vi "Cal Aux Corrections.vi"(8 "error in (no error)":errorcluster, 10 "Spectral distribution In":cluster{dbl, dbl}[](graph), 11 "Hardware Resources in":T1) -> (0 "error out":errorcluster, 2 "Spectral distribution Out":cluster{dbl, dbl}[](graph), 3 "Hardware Resources out":T1)   [LabVIEW 2013, in "AvaSpec.lvlib" / "AvaSpec Acquisition.lvlib"]
uses:
  AvaSpec Acquisition.lvlib
  Hardware Configuration.ctl
  Libraries/AS-5216-DLL/AVS settings.ctl
  Sphere Indicator.ctl
  Settings/Measurement Type.ctl
  AvaSpec.lvlib
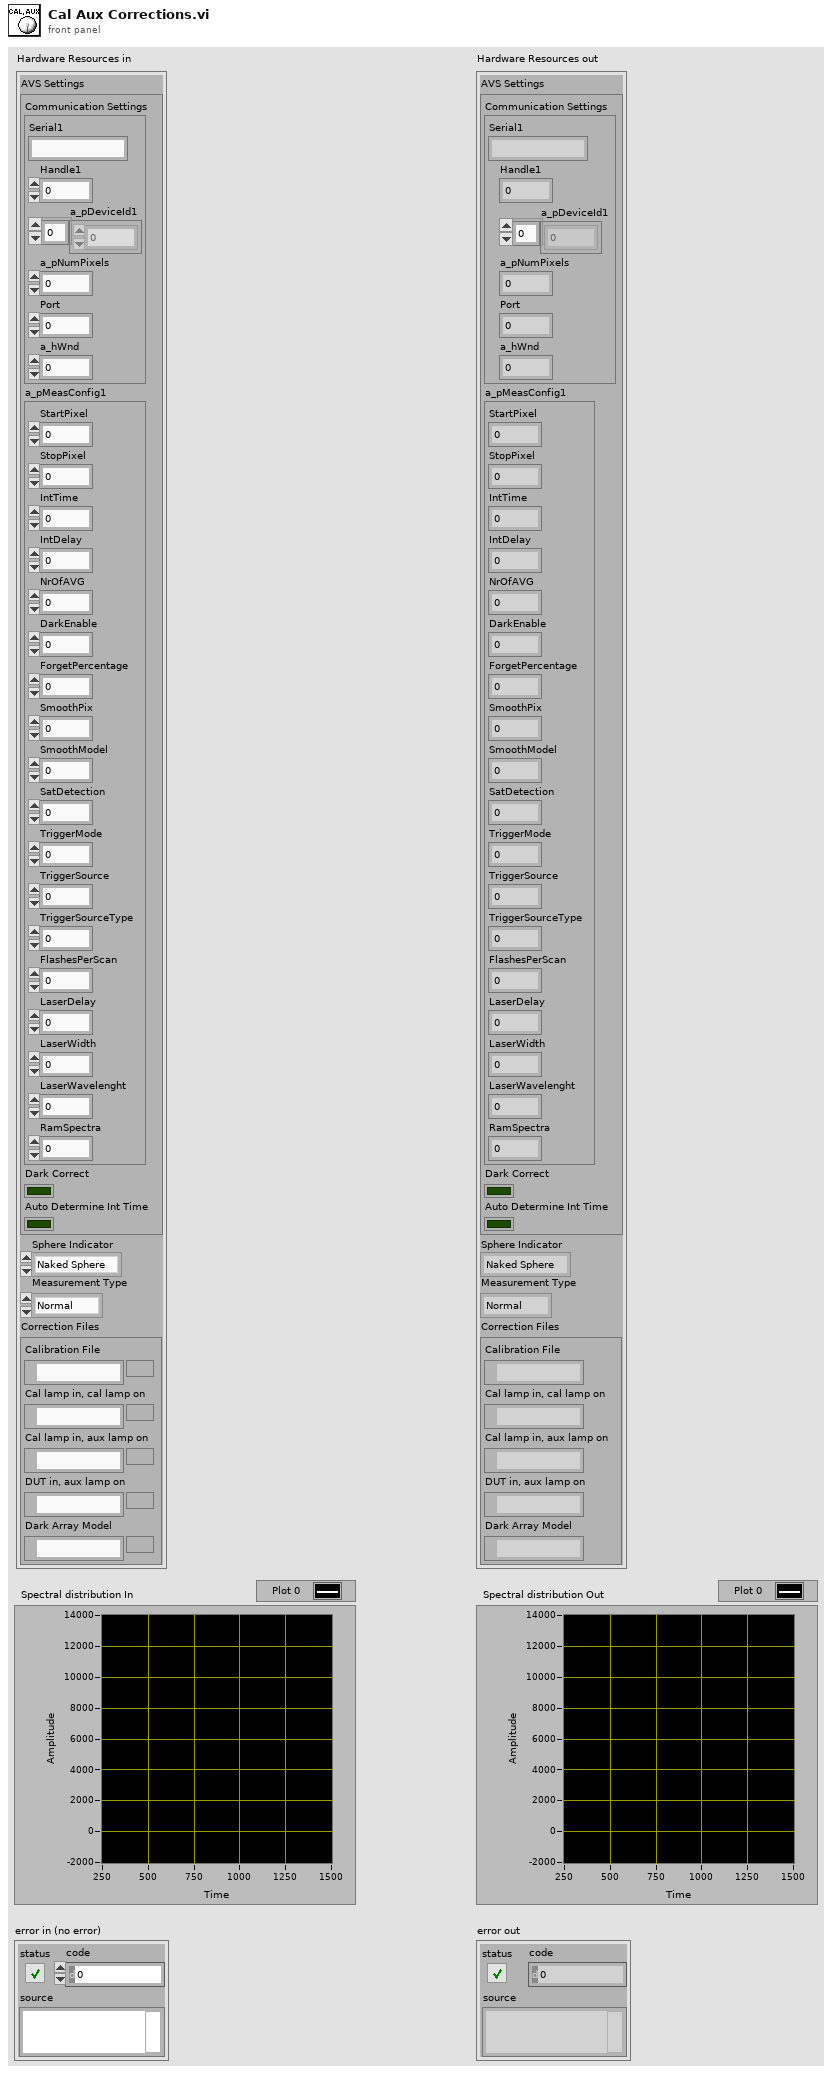
[diagram p1: front panel]
types:
  T1 = typedef "AvaSpec.lvlib/AvaSpec Acquisition.lvlib/Hardware Configuration.ctl" = cluster{"AVS Settings":T2, "Sphere Indicator":T3, "Measurement Type":T4, "Correction Files":cluster{"Calibration File":path, "Cal lamp in, cal lamp on":path, "Cal lamp in, aux lamp on":path, "DUT in, aux lamp on":path, "Dark Array Model":path}}
  T2 = typedef "AvaSpec.lvlib/AVS settings.ctl" = cluster{"Communication Settings":cluster{"Serial1":string, "Handle1":i32, "a_pDeviceId1":u8[], "a_pNumPixels":u16, "Port":i32, "a_hWnd":i32}, "a_pMeasConfig1":cluster{"StartPixel":u16, "StopPixel":u16, "IntTime":sgl, "IntDelay":u32, "NrOfAVG":u32, "DarkEnable":u8, "ForgetPercentage":u8, "SmoothPix":u16, "SmoothModel":u8, "SatDetection":u8, "TriggerMode":u8, "TriggerSource":u8, "TriggerSourceType":u8, "FlashesPerScan":u16, "LaserDelay":u32, "LaserWidth":u32, "LaserWavelenght":sgl, "RamSpectra":u16}, "Dark Correct":bool, "Auto Determine Int Time":bool}
  T3 = typedef "AvaSpec.lvlib/Sphere Indicator.ctl" = enum16{"Naked Sphere", "Insulated Sphere"}
  T4 = typedef "AvaSpec.lvlib/AvaSpec Acquisition.lvlib/Measurement Type.ctl" = enum16{"Normal", "Calibration", "Dark"}
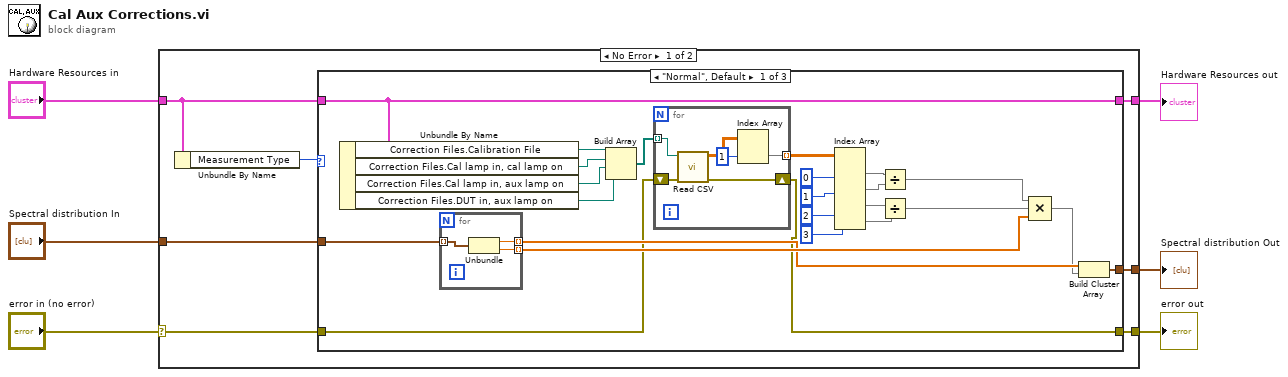
[diagram p0: block diagram]
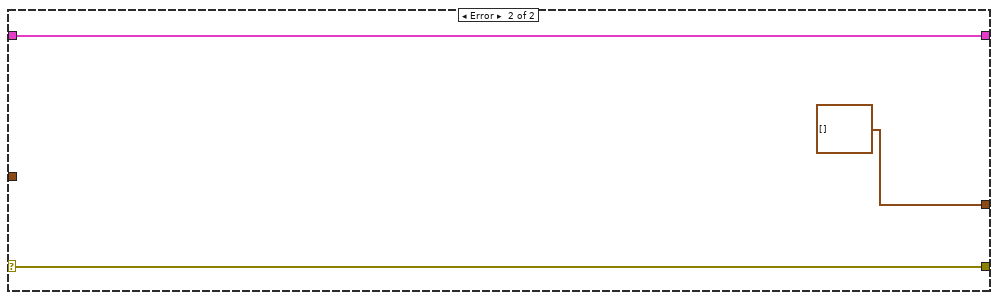
[diagram p4: hidden frame]
diagram:
  n1 = case shown="No Error" "error in (no error)" {
    selector: "error in (no error)" -> [w8 w55]
    tunnel: [w7 w55] -> w5
    tunnel: "Spectral distribution In" -> [w13 _]
    tunnel: "Hardware Resources in" -> [w11 w54]
    tunnel: [w9 w54] -> w2
    tunnel: [w12 cluster{dbl, dbl}[] [] ("Spectral distribution 3")] -> w1
    frame No Error {
      n2 = Unbundle By Name(w11) -> ("Measurement Type"=w10:T4)
      n3 = case shown="\"Normal\", Default" w10 {
        tunnel: w13 -> [w32 w48 w51]
        tunnel: [w23 w48 w51] -> w12
        tunnel: w11 -> [w22 w49 w52]
        tunnel: [w22 w49 w52] -> w9
        tunnel: w8 -> [w15 w47 w50]
        tunnel: [w14 w47 w50] -> w7
        frame "Normal", Default {
          n4 = Unbundle By Name(w22) -> ("Correction Files.Calibration File"=w37:path, "Correction Files.Cal lamp in, cal lamp on"=w36:path, "Correction Files.Cal lamp in, aux lamp on"=w35:path, "Correction Files.DUT in, aux lamp on"=w34:path)
          n5 = for {
            tunnel: w32 -> [w40] mode=indexing
            tunnel: [w39] -> w26 mode=indexing
            tunnel: [w38] -> w25 mode=indexing
            n6 = Unbundle(w40) -> (w38:dbl, w39:dbl)
          }
          n7 = Build Array(w37, w36, w35, w34) -> (w33:path[])
          n8 = for {
            tunnel: w33 -> [w44] mode=indexing
            tunnel: [w45] -> w31 mode=indexing
            shift-right: [w42] -> w14
            shift-left: w15 -> [w41]
            n9 = call "Read CSV.vi"("error in (no error)"=w41, "Path"=w44) -> ("error out"=w42:errorcluster, "all rows"=w43:dbl[][])  [unwired: 7 in, 1 out]
            n10 = Index Array(array=w43, index (col)=1 ("disabled index (col)")) -> (element=w45:dbl[])  [unwired: 1 in]
          }
          n11 = Index Array(array=w31, index (col) #1=0 ("disabled index (col)"), index (col) #2=1 ("index (col)"), index (col) #3=2 ("index (col)"), index (col) #4=3 ("index (col)")) -> (element #1=w21:dbl[], element #2=w20:dbl[], element #3=w19:dbl[], element #4=w18:dbl[])  [unwired: 4 in]
          n12 = Divide(x=w21, y=w20) -> (x/y=w17:dbl[])
          n13 = Divide(x=w19, y=w18) -> (x/y=w16:dbl[])
          n14 = Compound Arithmetic op=MULTIPLY(w17, w16, w26) -> (w24:dbl[])
          n15 = Build Cluster Array(w25, w24) -> (w23:cluster{dbl, dbl}[])
        }
        frame "Calibration" {
        }
        frame "Dark" {
        }
      }
    }
    frame Error {
    }
  }
  "error out" <- w5
  "Hardware Resources out" <- w2
  "Spectral distribution Out" <- w1
